vi "Shutdown.vi"(8 "error in (no error)":errorcluster, 10 "Kill Now? (T)":bool=TRUE, 11 "DbMeasurement in":refnum<class "DbMeasurement.lvclass">) -> (0 "error out":errorcluster, 3 "DbMeasurement out":refnum<class "DbMeasurement.lvclass">)   [LabVIEW 2013, in "DbMeasurement.lvclass"]
doc: "This method shuts down the measurement class, releasing the queue (which kills the asynchronous write data process), and closing the database file. By default, it waits until the queue is empty to release it. This can be overwritten with a Boolean input. This VI executes normally even if an error occurs before hand."
uses:
  DbMeasurement.lvclass
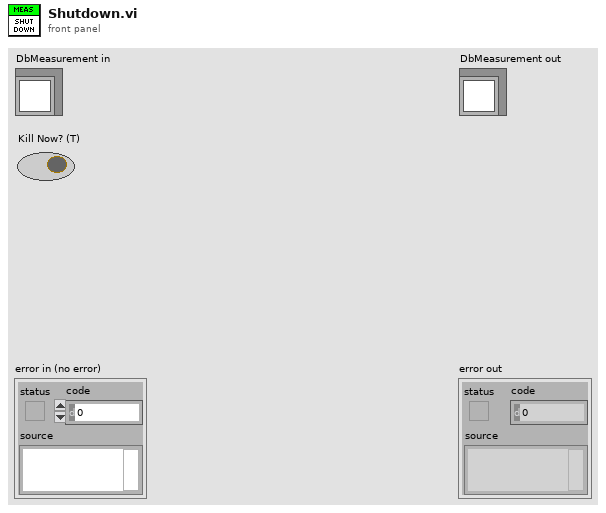
[diagram p1: front panel]
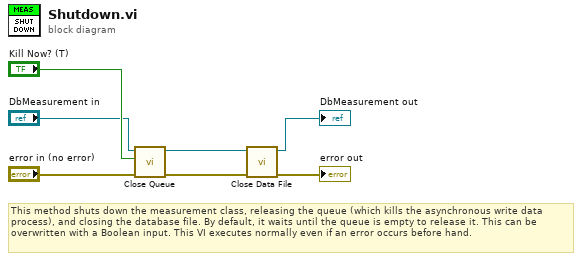
[diagram p0: block diagram]
diagram:
  # "This method shuts down the measurement class, releasing the queue (which kills the asynchronous write data process), and closing the database file. By default, it waits until the queue is empty to release it. This can be overwritten with a Boolean input. This VI executes normally even if an error occurs before hand."
  n1 = call "Close Queue.vi"("error in (no error)"="error in (no error)", "Kill Now? (T)"="Kill Now? (T)", "DbMeasurement in"="DbMeasurement in") -> ("error out"=w4:errorcluster, "DbMeasurement out"=w3:refnum<class "DbMeasurement.lvclass">)  [unwired: 7 in]
  n2 = call "Close Data File.vi"("error in (no error)"=w4, "DbMeasurement in"=w3) -> ("error out"=→"error out":errorcluster, "DbMeasurement out"=→"DbMeasurement out":refnum<class "DbMeasurement.lvclass">)  [unwired: 8 in]
